vi "AlazarOCTIgnoreBadClock.vi"(0 "Handle":u64, 5 "Enable":u32, 7 "Good Clock Duration":dbl, 9 "Bad Clock Duration":dbl, 11 "error in (no error)":errorcluster) -> (4 "Handle":u64, 6 "Trigger Cycle Time":dbl, 8 "Trigger Pulse Width":dbl, 10 "Return Code":u32, 15 "error out":errorcluster)   [LabVIEW 2018]
doc: "Get a board model identifier of the board associated with a board handle."
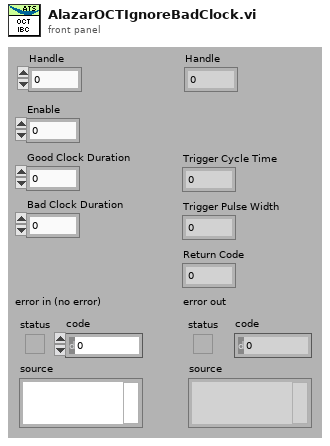
[diagram p1: front panel]
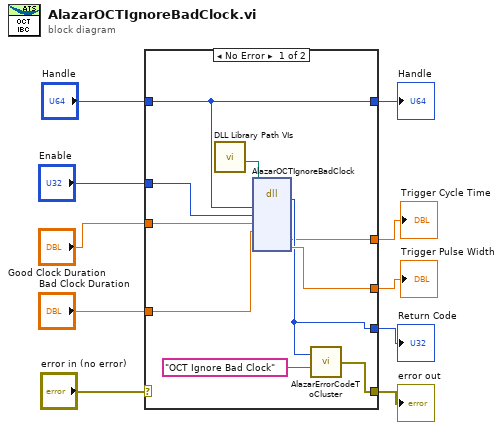
[diagram p0: block diagram]
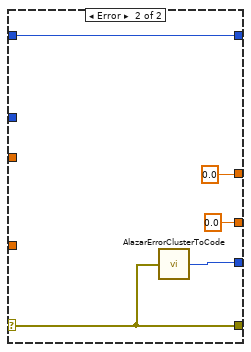
[diagram p2: hidden frame]
diagram:
  n1 = case shown="No Error" "error in (no error)" {
    selector: "error in (no error)" -> [_ w25]
    tunnel: [w14 w25] -> w9
    tunnel: [w13 w24] -> w8
    tunnel: "Handle" -> [w20 w23]
    tunnel: [w20 w23] -> w6
    tunnel: "Enable" -> [w19 _]
    tunnel: "Good Clock Duration" -> [w18 _]
    tunnel: "Bad Clock Duration" -> [w17 _]
    tunnel: [w16 0.0] -> w2
    tunnel: [w12 0.0] -> w1
    frame No Error {
      n2 = call "DLL Library Path VIs.vi"() -> ("Alazar"=w11:path)  [unwired: 9 in, 2 out]
      n3 = dll-call lib="C:/Project/SerialSectOCT - FFT GPU/SerialSectOCT/Labview Software/DLL/ATSApi.dll" fn="AlazarOCTIgnoreBadClock"(path in=w11, "handle"=w20, "enable"=w19, "goodClockDuration"=w18, "badClockDuration"=w17) -> ("return type"=w13:u32, "triggerCycleTime"=w12:dbl, "triggerPulseWidth"=w16:dbl)  [unwired: 8 in, 2 out]
      n4 = call "AlazarErrorCodeToCluster.vi"("Message"="OCT Ignore Bad Clock", "Error Code"=w13) -> ("error out"=w14:errorcluster)
    }
    frame Error {
      n5 = call "AlazarErrorClusterToCode.vi"("error in (no error)"=w25) -> ("Error Code"=w24:u32)
    }
  }
  "Handle" <- w6
  "error out" <- w9
  "Return Code" <- w8
  "Trigger Cycle Time" <- w1
  "Trigger Pulse Width" <- w2
